vi "CreatePublicEvents.vi"(8 "error in (no error)":errorcluster, 11 "ZMQ":refnum<class "ZMQ_SMO.lvclass">) -> (0 "error out":errorcluster, 3 "ZMQ out":refnum<class "ZMQ_SMO.lvclass">)   [LabVIEW 2016, in "ZMQ_SMO.lvclass"]
doc: "---------------------------------------------------------------\nJKI State Machine Objects™\nhttp://jki.net/state-machine-objects/\nCopyright (C) 2005-2015, JKI <info@jki.net>\nALL RIGHTS RESERVEDJKI State Machine Objects (SMO) 1.0.0.4\nJKI - JKI\nCopyright (c) 2015, JKI"
uses:
  ZMQ_SMO.lvclass
  Typedefs/PublicEvents--ZMQ.ZMQ_PublicEvent.ctl
  ZMQ_SMO.lvclass/ZMQ_SMO.ctl
  <vilib>/JKI/JKI SMO/SMO/SMO.lvclass
panel:
  # "For instructions on how to use the JKI State Machine Objects, examples and video tutorials, visit:\nhttp://jki.net/state-machine-objects/\n\nJKI State Machine Objects™\nhttp://jki.net/state-machine-objects/\nCopyright (C) 2005-2015, JKI <info@jki.net>\nALL RIGHTS RESERVED"
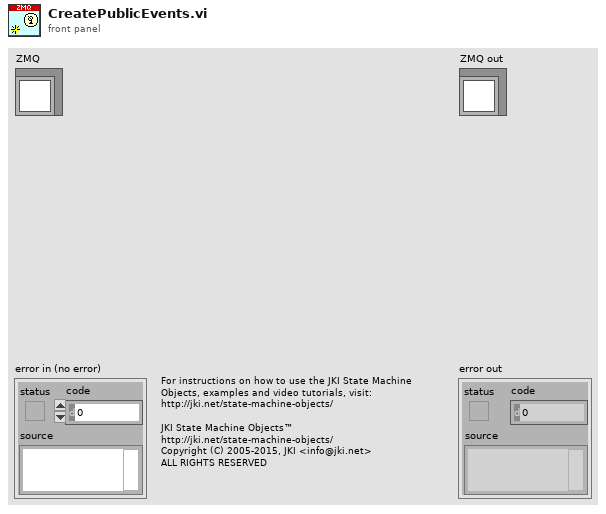
[diagram p1: front panel]
types:
  T1 = typedef "ZMQ_SMO.lvclass/PublicEvents--ZMQ.ZMQ_PublicEvent.ctl" = string[]
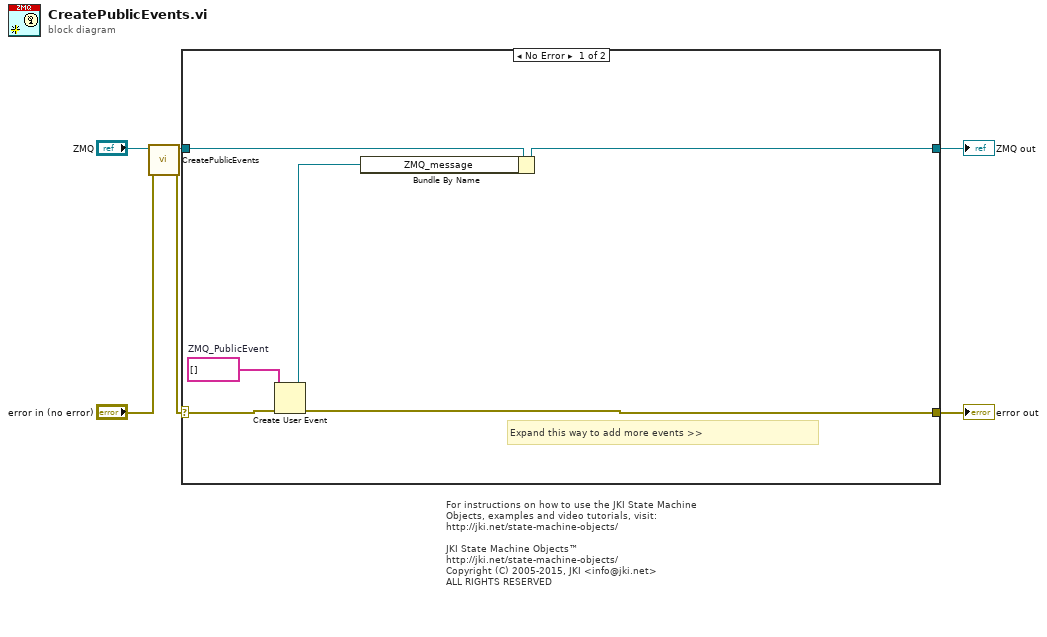
[diagram p0: block diagram]
diagram:
  # "For instructions on how to use the JKI State Machine Objects, examples and video tutorials, visit:\nhttp://jki.net/state-machine-objects/\n\nJKI State Machine Objects™\nhttp://jki.net/state-machine-objects/\nCopyright (C) 2005-2015, JKI <info@jki.net>\nALL RIGHTS RESERVED"
  n1 = call-parent "CreatePublicEvents.vi"("error in (no error)"="error in (no error)", "SMO"="ZMQ") -> ("error out"=w1:errorcluster, "SMO out"=w3:refnum<class "ZMQ_SMO.lvclass">)  [unwired: 8 in]
  n2 = case shown="No Error" w1 {
    selector: w1 -> [w11 w14]
    tunnel: [w9 w14] -> w5
    tunnel: [w10 w13] -> w6
    tunnel: w3 -> [w12 w13]
    frame No Error {
      w8 = T1 []  # ZMQ_PublicEvent
      # "Expand this way to add more events >>"
      n3 = Create User Event(user event datatype=w8, error in=w11) -> (user event=w7:refnum<user-event>, error out=w9:errorcluster)
      n4 = Bundle By Name(cluster=w12, "ZMQ_message"=w7) -> (w10:refnum<class "ZMQ_SMO.lvclass">)
    }
    frame Error {
    }
  }
  "error out" <- w5
  "ZMQ out" <- w6
